vi "Get_RT_Queue.vi"(11 "String":string) -> (1 "rt fifo boolean":refnum<k33>, 2 "rt fifo double":refnum<k33>, 3 "rt fifo single":refnum<k33>)   [LabVIEW 2020]
panel:
  out "error out":errorcluster
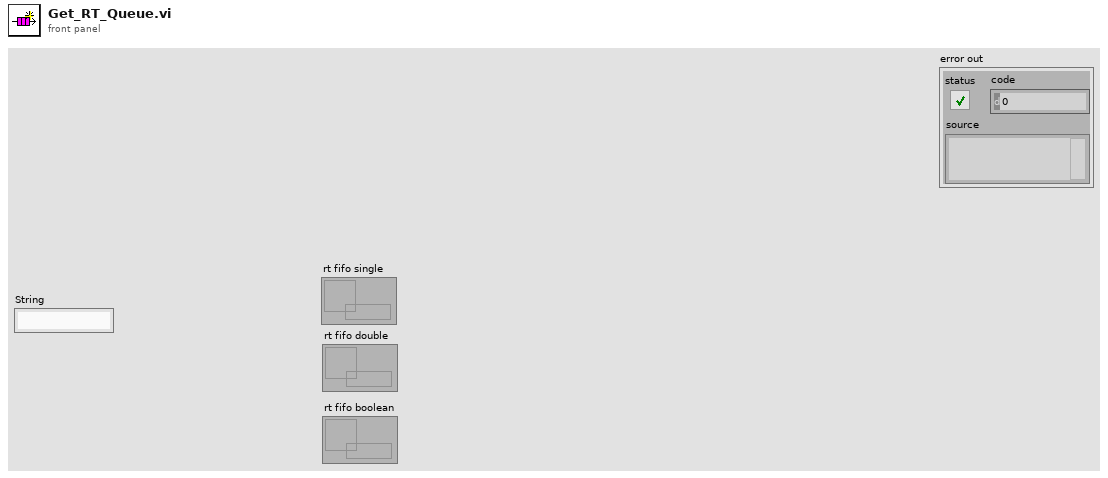
[diagram p1: front panel]
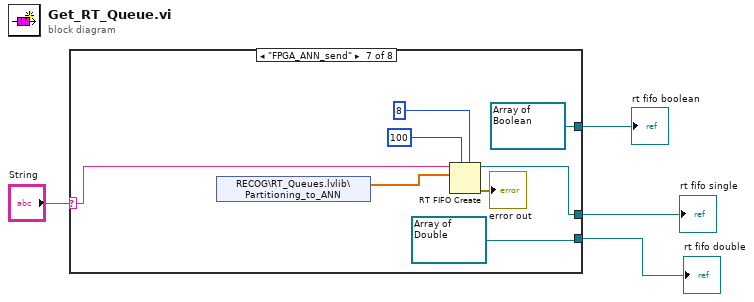
[diagram p0: block diagram]
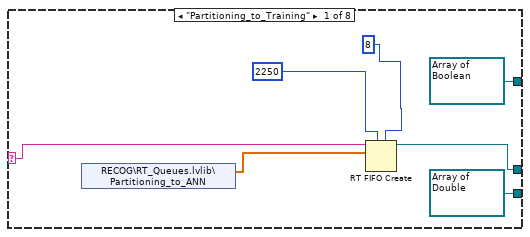
[diagram p2: hidden frame]
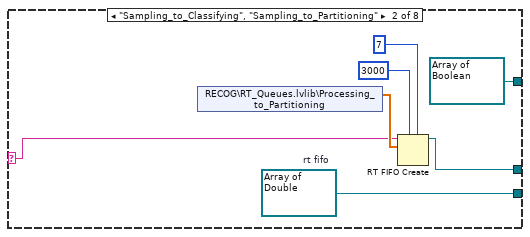
[diagram p3: hidden frame]
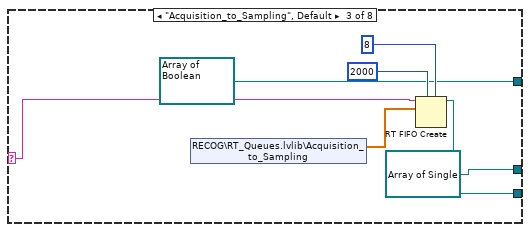
[diagram p4: hidden frame]
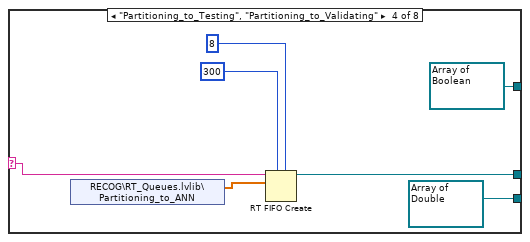
[diagram p5: hidden frame]
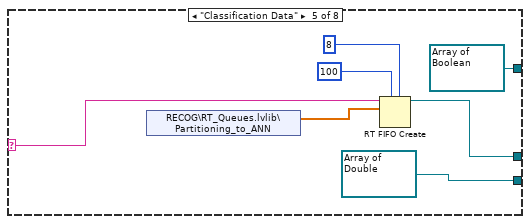
[diagram p6: hidden frame]
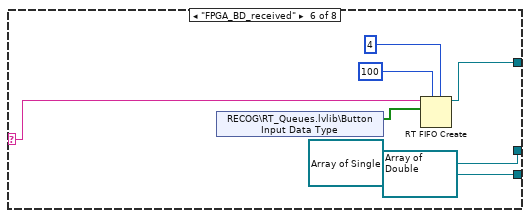
[diagram p7: hidden frame]
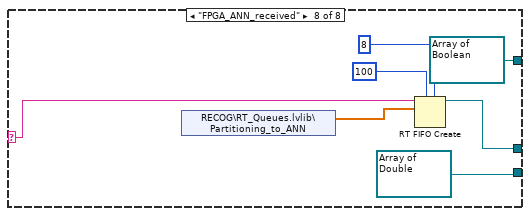
[diagram p8: hidden frame]
diagram:
  n1 = case shown="\"FPGA_ANN_send\"" "String" {
    selector: "String" -> [w10 w17 w24 w29 w36 w44 w49 w56]
    tunnel: [w7 w14 refnum<k33> refnum ("rt fifo") w28 w35 refnum<k33> refnum ("rt fifo") w50 w57] -> w3
    tunnel: [refnum<k33> refnum ("rt fifo") w13 w21 refnum<k33> refnum ("rt fifo") refnum<k33> refnum ("rt fifo") refnum<k33> refnum ("rt fifo") refnum<k33> refnum ("rt fifo") refnum<k33> refnum ("rt fifo")] -> w2
    tunnel: [refnum<k33> refnum ("rt fifo") refnum<k33> refnum ("rt fifo") refnum<k33> refnum ("rt fifo") refnum<k33> refnum ("rt fifo") refnum<k33> refnum ("rt fifo") w42 refnum<k33> refnum ("rt fifo") refnum<k33> refnum ("rt fifo")] -> w1
    frame "Partitioning_to_Training" {
      n2 = shared-variable "RECOG\\RT_Queues.lvlib\\Partitioning_to_ANN"() -> (w11:sgl[])  [unwired: 1 in, 1 out]
      n3 = RT FIFO Create(0:w10, 1:w11, 4:u16 2250 ("port"), 6:u16 8 ("port")) -> (8:w7:refnum<k33>)  [unwired: 4 in, 2 out]
    }
    frame "Sampling_to_Classifying", "Sampling_to_Partitioning" {
      w13 = refnum<k33> refnum  # rt fifo
      n4 = shared-variable "RECOG\\RT_Queues.lvlib\\Processing_to_Partitioning"() -> (w18:sgl[])  [unwired: 1 in, 1 out]
      n5 = RT FIFO Create(0:w17, 1:w18, 4:u16 3000 ("port"), 6:u16 7 ("port")) -> (8:w14:refnum<k33>)  [unwired: 4 in, 2 out]
    }
    frame "Acquisition_to_Sampling", Default {
      n6 = shared-variable "RECOG\\RT_Queues.lvlib\\Acquisition_to_Sampling"() -> (w25:dbl[])  [unwired: 1 in, 1 out]
      n7 = RT FIFO Create(0:w24, 1:w25, 4:u16 2000 ("port"), 6:u16 8 ("port")) -> (8:w21:refnum<k33>)  [unwired: 4 in, 2 out]
    }
    frame "Partitioning_to_Testing", "Partitioning_to_Validating" {
      n8 = shared-variable "RECOG\\RT_Queues.lvlib\\Partitioning_to_ANN"() -> (w30:sgl[])  [unwired: 1 in, 1 out]
      n9 = RT FIFO Create(0:w29, 1:w30, 4:u16 300 ("port"), 6:u16 8 ("port")) -> (8:w28:refnum<k33>)  [unwired: 4 in, 2 out]
    }
    frame "Classification Data" {
      n10 = shared-variable "RECOG\\RT_Queues.lvlib\\Partitioning_to_ANN"() -> (w39:sgl[])  [unwired: 1 in, 1 out]
      n11 = RT FIFO Create(0:w36, 1:w39, 4:u16 100 ("port"), 6:u16 8 ("port")) -> (8:w35:refnum<k33>)  [unwired: 4 in, 2 out]
    }
    frame "FPGA_BD_received" {
      n12 = shared-variable "RECOG\\RT_Queues.lvlib\\Button Input Data Type"() -> (w43:bool[])  [unwired: 1 in, 1 out]
      n13 = RT FIFO Create(0:w44, 1:w43, 4:u16 100 ("port"), 6:u16 4 ("port")) -> (8:w42:refnum<k33>)  [unwired: 4 in, 2 out]
    }
    frame "FPGA_ANN_send" {
      n14 = shared-variable "RECOG\\RT_Queues.lvlib\\Partitioning_to_ANN"() -> (w54:sgl[])  [unwired: 1 in, 1 out]
      n15 = RT FIFO Create(0:w49, 1:w54, 4:u16 100 ("port"), 6:u16 8 ("port")) -> (8:w50:refnum<k33>, 11:→"error out":errorcluster)  [unwired: 4 in, 1 out]
    }
    frame "FPGA_ANN_received" {
      n16 = shared-variable "RECOG\\RT_Queues.lvlib\\Partitioning_to_ANN"() -> (w61:sgl[])  [unwired: 1 in, 1 out]
      n17 = RT FIFO Create(0:w56, 1:w61, 4:u16 100 ("port"), 6:u16 8 ("port")) -> (8:w57:refnum<k33>)  [unwired: 4 in, 2 out]
    }
  }
  "rt fifo single" <- w3
  "rt fifo double" <- w2
  "rt fifo boolean" <- w1
